vi "One note refresh.vi"(8 "error in":errorcluster, 9 "Refresh Token In":string, 11 "Authorization Code In":string) -> (0 "error out":errorcluster, 1 "Refresh Token Out":string, 2 "Access Token Out":string, 3 "Auth Code Out":string)   [LabVIEW 2016]
uses:
  <vilib>/httpClient/POSTBuffer.vi
  <vilib>/httpClient/LabVIEWHTTPClient.lvlib
  <vilib>/addons/_JKI.lib/Serialization/JSON/JKI JSON Serialization.lvlib
  Object Oriented Version/Response/Response.lvclass
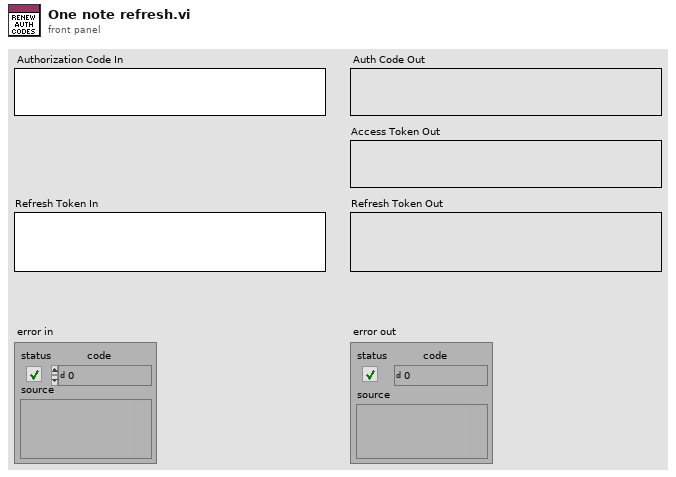
[diagram p1: front panel]
types:
  T1 = cluster{"token_type":string, "scope":string, "access_token":string, "refresh_token":string, "user_id":string, "expires_in":i32}
  T2 = typedef "LabVIEWHTTPClient.lvlib/ClientHandle.ctl" = refnum<k1>
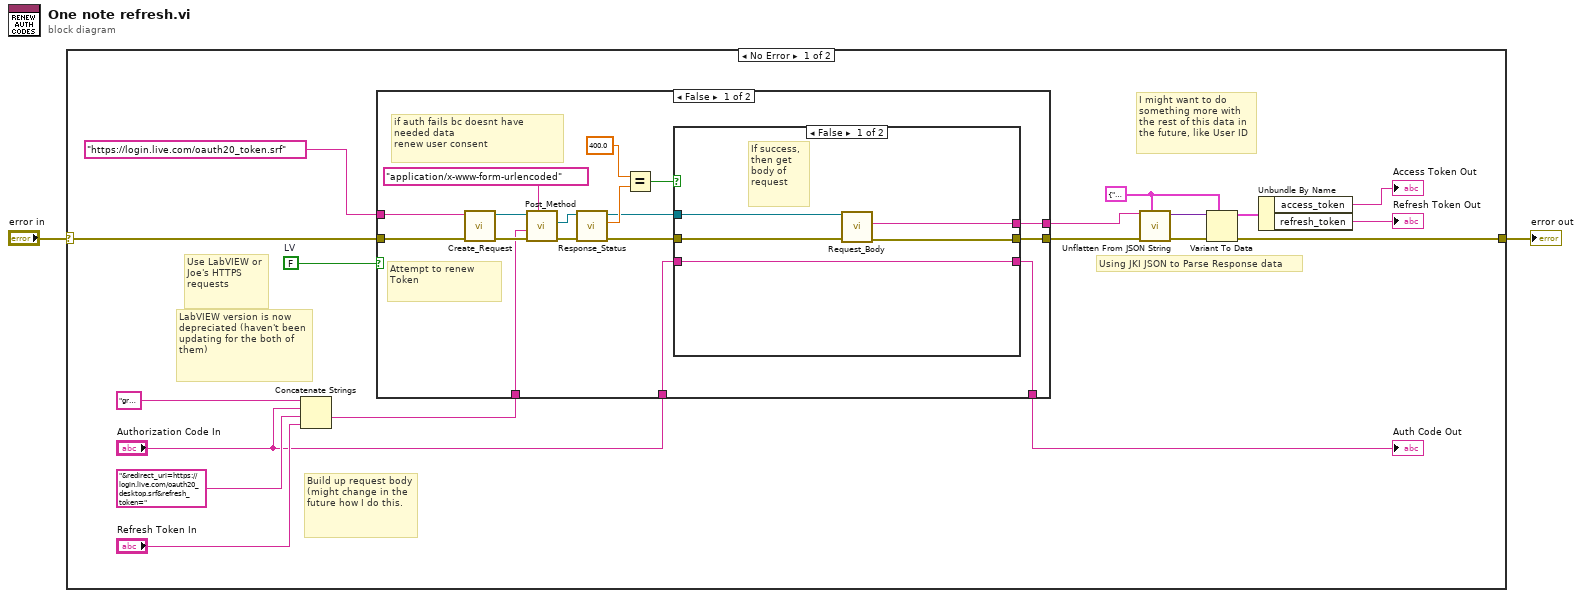
[diagram p0: block diagram]
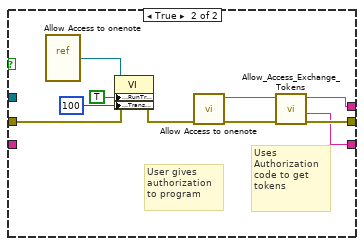
[diagram p2: hidden frame]
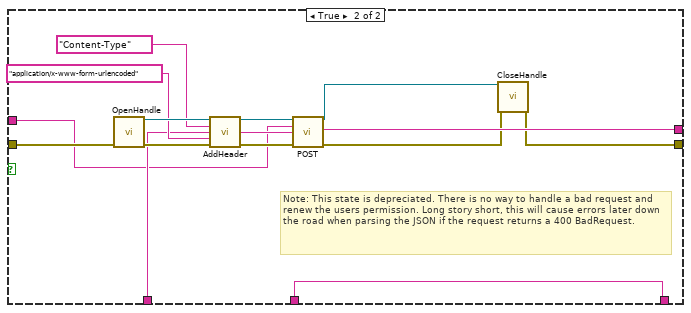
[diagram p3: hidden frame]
diagram:
  n1 = case shown="No Error" "error in" {
    selector: "error in" -> [w13 w67]
    tunnel: [w14 w67] -> w1
    frame No Error {
      w6 = T1 {"token_type"="", "scope"="", "access_token"="", "refresh_token"="", "user_id"="", "expires_in"=0}
      w9 = FALSE  # LV
      # "LabVIEW version is now depreciated (haven't been updating for the both of them)"
      # "Use LabVIEW or Joe's HTTPS requests"
      # "Build up request body (might change in the future how I do this."
      # "I might want to do something more with the rest of this data in the future, like User ID"
      # "Using JKI JSON to Parse Response data"
      n2 = Concatenate Strings("grant_type=refresh_token&client_id=c698ce01-75b1-4eb8-b040-9787b75e6b48&code=" ("string"), "Authorization Code In", "&redirect_uri=https://login.live.com/oauth20_desktop.srf&refresh_token=", "Refresh Token In") -> (w8:string)
      n3 = case shown="False" w9 {
        tunnel: [w26 w62] -> w17
        tunnel: [w28 w54] -> w16
        tunnel: w13 -> [w35 w59]
        tunnel: "https://login.live.com/oauth20_token.srf" ("url") -> [w36 w56]
        tunnel: "Authorization Code In" -> [w24 w57]
        tunnel: [w23 w57] -> w10
        tunnel: w8 -> [w22 w58]
        frame False {
          # "Attempt to renew Token"
          # "if auth fails bc doesnt have needed data\nrenew user consent"
          n4 = call "Create_Request.vi"("error in (no error)"=w35, "Base URL"=w36) -> ("error out"=w34:errorcluster, "Request out"=w37:refnum<class "Request.lvclass">)  [unwired: 8 in]
          n5 = call "Post_Method.vi"("Body Content-Type"="application/x-www-form-urlencoded", "error in (no error)"=w34, "Body"=w22, "Request in"=w37) -> ("error out"=w33:errorcluster, "Response out"=w32:refnum<class "Response.lvclass">)  [unwired: 5 in, 1 out]
          n6 = call "Response_Status.vi"("error in (no error)"=w33, "Response in"=w32) -> ("error out"=w29:errorcluster, "Status Code"=w31:dbl, "Response out"=w25:refnum<class "Response.lvclass">)  [unwired: 6 in, 1 out]
          n7 = Equal?(x=400.0, y=w31) -> (x = y?=w27:bool)
          n8 = case shown="False" w27 {
            tunnel: [w41 w50] -> w28
            tunnel: w29 -> [w42 w44]
            tunnel: [w39 w48] -> w26
            tunnel: w25 -> [w40 _]
            tunnel: w24 -> [w38 _]
            tunnel: [w38 w49] -> w23
            frame False {
              # "If success, then get body of request"
              n9 = call "Request_Body.vi"("error in (no error)"=w42, "Response in"=w40) -> ("error out"=w41:errorcluster, "Response Body"=w39:string)  [unwired: 7 in, 1 out]
            }
            frame True {
              # "Uses Authorization code to get tokens"
              # "User gives authorization to program"
              n10 = vi-ref "Allow Access to onenote.vi"() -> (w47:refnum<vi>)
              n11 = property class="VI"(reference=w47, error in=w44, "FP:RunTransparently"=TRUE ("Front Panel Window:Run VI Transparently"), "FP:Transparency"=u8 100 ("Front Panel Window:Transparency")) -> (error out=w43:errorcluster)  [unwired: 1 out]
              n12 = call "Allow Access to onenote.vi"("error in (no error)"=w43) -> ("error out"=w51:errorcluster, "LocationURL"=w52:string)  [unwired: 9 in]
              n13 = call "Allow_Access_Exchange_Tokens.vi"("error in (no error)"=w51, "Location URL"=w52) -> ("error out"=w50:errorcluster, "Authorization Code"=w49:string, "body"=w48:string)  [unwired: 7 in]
            }
          }
        }
        frame True {
          # "Note: This state is depreciated. There is no way to handle a bad request and renew the users permission. Long story short, this will cause errors later down the road when parsing the JSON if the request returns a 400 BadRequest."
          n14 = call <vilib>:"OpenHandle.vi"("error in (no error)"=w59) -> ("client handle out"=w66:T2, "error out"=w61:errorcluster)  [unwired: 13 in]
          n15 = call <vilib>:"AddHeader.vi"("client handle"=w66, "header"="Content-Type", "value"="application/x-www-form-urlencoded", "error in (no error)"=w61) -> ("client handle out"=w63:T2, "error out"=w60:errorcluster)  [unwired: 10 in]
          n16 = call-poly <vilib>:"POST.vi"("client handle"=w63, "url"=w56, "buffer"=w58, "error in (no error)"=w60) -> ("client handle out"=w53:T2, "body"=w62:string, "error out"=w55:errorcluster)  [unwired: 8 in, 1 out]
          n17 = call <vilib>:"CloseHandle.vi"("client handle"=w53, "error in (no error)"=w55) -> ("error out"=w54:errorcluster)  [unwired: 13 in]
        }
      }
      "Auth Code Out" <- w10
      n18 = call <vilib>:"Unflatten From JSON String.vi"("Type and Defaults"=w6, "error in (no error)"=w16, "JSON String"=w17) -> ("error out"=w7:errorcluster, "Variant"=w5:variant)  [unwired: 7 in]
      n19 = Variant To Data(error in=w7, type=w6, Variant=w5) -> (data=w4:T1, error out=w14:errorcluster)
      n20 = Unbundle By Name(w4) -> ("access_token"=→"Access Token Out":string, "refresh_token"=→"Refresh Token Out":string)
    }
    frame Error {
    }
  }
  "error out" <- w1
